vi "Begin.vi"(8 "error in":errorcluster) -> (0 "error out":errorcluster)   [LabVIEW 2019]
doc: "Called before other user functions, this VI is expected to open initial I/O refnums, load in file data, and do all program initialization. Notice that the <B>error out</B> terminal is simply used for data flow. Wiring it to other structures or subVIs ensures that this VI runs first."
uses:
  <vilib>/Rock Robotics/WPI/DriverStation/WPI_DriverStationRobotMode2.ctl
  <vilib>/Rock Robotics/WPI/Joystick/WPI_JoystickDeviceEnum.ctl
  <vilib>/Rock Robotics/SystemInterfaces/DIO/FPGA_DIOPWMChannel.ctl
  <vilib>/Rock Robotics/SystemInterfaces/DIO/FPGA_DIORelayChannel.ctl
  <vilib>/Rock Robotics/WPI/Solenoid/WPI_SolenoidChannel.ctl
  <vilib>/Rock Robotics/SystemInterfaces/DIO/FPGA_DIOChannel.ctl
  <vilib>/Rock Robotics/SystemInterfaces/i2clib/i2c_bus.ctl
  <vilib>/Rock Robotics/SystemInterfaces/AI/FPGA_AIChannel.ctl
  <vilib>/Rock Robotics/SystemInterfaces/spilib/spi_bus.ctl
  Robot Global Data.vi
  <vilib>/Rock Robotics/WPI/MotorControl/WPI_MotorControlOpen SPARK.vi
  <vilib>/Rock Robotics/WPI/MotorControl/WPI_MotorControlOpen Talon.vi
  <vilib>/Rock Robotics/WPI/Solenoid/WPI_SolenoidOpenSingle.vi
  <vilib>/Rock Robotics/WPI/Counter/WPI_CounterDigitalInputToDigitalSource.vi
  Program Files/navX.Library.v2/navX Library v2/IO/Open/Z900_navX_Open_SPI.vi
  Program Files/navX.Library.v2/navX Library v2/navX Library v2.lvlib
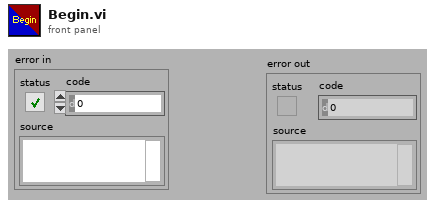
[diagram p1: front panel]
types:
  T1 = typedef "WPI_DriverStationRobotMode2.ctl" = enum16{"Autonomous Disabled", "Autonomous Enabled", "Teleop Disabled", "Teleop Enabled", "Disconnected", "Finish", "Test Disabled", "Test Enabled", "Emergency Stopped"}
  T2 = typedef "WPI_JoystickDeviceEnum.ctl" = enum16{"USB 0", "USB 1", "USB 2", "USB 3", "USB 4", "USB 5"}
  T3 = typedef "WPI_SolenoidChannel.ctl" = enum8{"Solenoid 0", "Solenoid 1", "Solenoid 2", "Solenoid 3", "Solenoid 4", "Solenoid 5", "Solenoid 6", "Solenoid 7", "Invalid"}
  T4 = typedef "FPGA_DIORelayChannel.ctl" = enum8{"Relay 0", "Relay 1", "Relay 2", "Relay 3", "Invalid"}
  T5 = typedef "FPGA_DIOPWMChannel.ctl" = enum8{"PWM 0", "PWM 1", "PWM 2", "PWM 3", "PWM 4", "PWM 5", "PWM 6", "PWM 7", "PWM 8", "PWM 9", "PWM MXP 0", "PWM MXP 1", "PWM MXP 2", "PWM MXP 3", "PWM MXP 4", "PWM MXP 5", "PWM MXP 6", "PWM MXP 7", "PWM MXP 8", "PWM MXP 9", "Invalid"}
  T6 = typedef "FPGA_AIChannel.ctl" = enum8{"AI 0", "AI 1", "AI 2", "AI 3", "AI MXP 0", "AI MXP 1", "AI MXP 2", "AI MXP 3", "Invalid"}
  T7 = typedef "spi_bus.ctl" = enum16{"SPI On-Board, CS0", "SPI On-Board, CS1", "SPI On-Board, CS2", "SPI On-Board, CS3", "SPI MXP", "Invalid"}
  T8 = typedef "i2c_bus.ctl" = enum16{"I2C On-Board", "I2C MXP", "Invalid"}
  T9 = typedef "WPI_CompressorDevRef.ctl" = cluster{"DevStatus":errorcluster, "Pneumatics Control Module":u8}
  T10 = typedef "WPI_JoystickDevRef.ctl" = cluster{"Device":T2}
  T11 = typedef "WPI_MotorControlDeviceRef.ctl" = cluster{"DeviceStatus":errorcluster, "Type":T12, "PWM":cluster{"PWM Channel":T5, "DeadBand":T13}, "CAN":cluster{"Device Number":u8, "SetOutput VI Ref":variant, "GetOutput VI Ref":variant, "Enable VI Ref":variant, "Disable VI Ref":variant, "Data":variant}, "Invert":bool, "DIO PWM":cluster{"PWM \"Enable\" Channel":T5, "DIOChannel":T14, "PWM Rate":dbl}}
  T12 = typedef "WPI_MotorControlType.ctl" = enum16{"PWM", "CAN", "DIO PWM"}
  T13 = typedef "WPI_PWMDeadband.ctl" = cluster{"Name":string, "maxPositivePwm":i32, "minPositivePwm":i32, "centerPwm":i32, "maxNegativePwm":i32, "minNegativePwm":i32, "angularRange":u16}
  T14 = typedef "FPGA_DIOChannel.ctl" = enum8{"DIO 0", "DIO 1", "DIO 2", "DIO 3", "DIO 4", "DIO 5", "DIO 6", "DIO 7", "DIO 8", "DIO 9", "DIO MXP 0", "DIO MXP 1", "DIO MXP 2", "DIO MXP 3", "DIO MXP 4", "DIO MXP 5", "DIO MXP 6", "DIO MXP 7", "DIO MXP 8", "DIO MXP 9", "DIO MXP 10", "DIO MXP 11", "DIO MXP 12", "DIO MXP 13", "DIO MXP 14", "DIO MXP 15", "SPI Port CS1", "SPI Port CS2", "SPI Port CS3", "SPI Port MISO", "SPI Port MOSI", "Invalid"}
  T15 = typedef "WPI_RelayDevRef.ctl" = cluster{"DevStatus":errorcluster, "Relay Channel":T4, "Relay Direction":T16}
  T16 = typedef "WPI_RelayDirection.ctl" = enum16{"Both directions", "Forward only", "Reverse only"}
  T17 = typedef "WPI_SolenoidDevRef.ctl" = cluster{"DevStatus":errorcluster, "Pneumatics Control Module":u8, "Forward Solenoid Channel":T3, "Reverse Solenoid Channel":T3}
  T18 = typedef "WPI_DigitalInputDevRef.ctl" = cluster{"DevStatus":errorcluster, "DIO Channel":T14}
  T19 = typedef "WPI_AnalogChannelDevRef.ctl" = cluster{"DevStatus":errorcluster, "Analog Channel":T6}
  T20 = typedef "navX Library v2.lvlib/Z900_navX_DeviceTypeDef.ctl" = cluster{"Interface":cluster{"Protocol":T21, "Update Rate (4Hz-100Hz)":u8, "navX Open TypeDef":variant}, "Notify Packet":refnum<notifier>, "Loop VI Refnum":refnum<vi>, "Ready to Close Occurrence Refnum":refnum<k4>}
  T21 = typedef "navX Library v2.lvlib/Z900_navX_ProtocolTypeDef.ctl" = enum16{"SERIAL", "I2C", "SPI"}
  T22 = typedef "FPGA_CounterEncoderSourceConvertionLVSourceType.ctl" = cluster{"DevStatus":errorcluster, "AnalogTriggerMode?":bool, "DigitalMode":cluster{"DIO Channel":T23}, "AnalogTriggerMode":cluster{"AnalogTriggerIndex":T24, "OutputType":T25}}
  T23 = typedef "FPGA_DIODigitalSourceChannel.ctl" = enum8{"DIO 0", "DIO 1", "DIO 2", "DIO 3", "DIO 4", "DIO 5", "DIO 6", "DIO 7", "DIO 8", "DIO 9", "DIO MXP 0", "DIO MXP 1", "DIO MXP 2", "DIO MXP 3", "DIO MXP 4", "DIO MXP 5", "DIO MXP 6", "DIO MXP 7", "DIO MXP 8", "DIO MXP 9", "DIO MXP 10", "DIO MXP 11", "DIO MXP 12", "DIO MXP 13", "DIO MXP 14", "DIO MXP 15", "SPI Port CS1", "SPI Port CS2", "SPI Port CS3", "SPI Port MISO", "SPI Port MOSI", "Disabled"}
  T24 = typedef "FPGA_AnalogTriggerIndex.ctl" = enum8{"Trig 0", "Trig 1", "Trig 2", "Trig 3", "Trig 4", "Trig 5", "Trig 6", "Trig 7", "Invalid"}
  T25 = typedef "FPGA_AnalogTriggerOutType.ctl" = enum16{"InWindow", "TriggerState", "Rising", "Falling"}
  T26 = typedef "Color Sensor V3 DevRef.ctl" = cluster{"I2CDevRef":T27}
  T27 = typedef "WPI_I2CDevRef.ctl" = cluster{"DevStatus":errorcluster, "Device Address":u8, "Handle":i32, "I2C Bus":T8}
  T28 = typedef "WPI_EncoderDevRef.ctl" = cluster{"DevStatus":errorcluster, "EncoderIndex":T29, "CounterIndex":T30, "DistancePerCount":dbl, "Decoding Type":T31}
  T29 = typedef "FPGA_EncoderIdx.ctl" = enum8{"Enc 0", "Enc 1", "Enc 2", "Enc 3", "Enc 4", "Enc 5", "Enc 6", "Enc 7", "Invalid"}
  T30 = typedef "FPGA_CounterCtrSystemIndex.ctl" = enum8{"Ctr 0", "Ctr 1", "Ctr 2", "Ctr 3", "Ctr 4", "Ctr 5", "Ctr 6", "Ctr 7", "Invalid"}
  T31 = typedef "WPI_EncoderType.ctl" = enum16{"1x", "2x", "4x"}
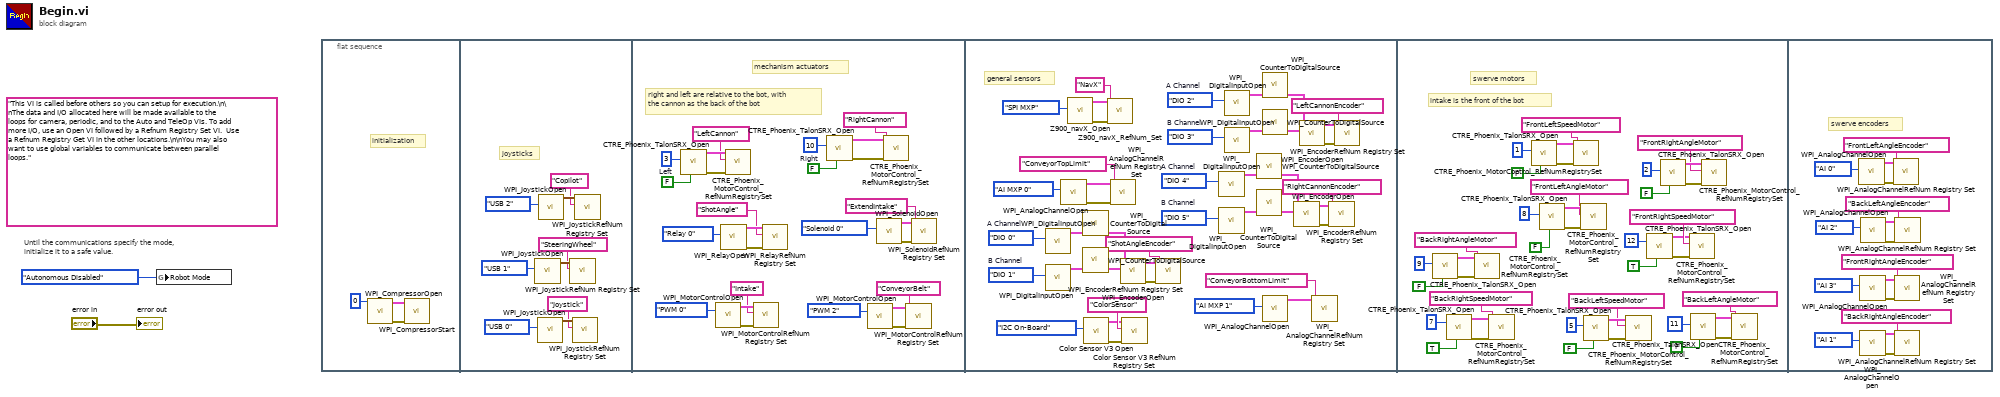
[diagram p0: block diagram]
diagram:
  (unwired) "This VI is called before others so you can setup for execution.\n\nThe data and I/O allocated here will be made available to the loops for camera, periodic, and to the Auto and TeleOp VIs. To add more I/O, use an Open VI followed by a Refnum Registry Set VI.  Use a Refnum Registry Get VI in the other locations.\n\nYou may also want to use global variables to communicate between parallel loops."
  # "Until the communications specify the mode,\ninitialize it to a safe value."
  n1 = global write "Robot Global Data.vi" "Robot Mode"(WPI_DriverStationRobotMode2."Autonomous Disabled" ("Robot Mode")) -> ()
  n2 = flat-sequence {
    frame #0 {
      # "initialization"
      n3 = call <vilib>:"WPI_CompressorOpen.vi"("Pneumatics Control Module (0)"=u8 0) -> ("CompressorDevRef"=w3:T9, "error out"=w5:errorcluster)  [unwired: 13 in]
      n4 = call <vilib>:"WPI_CompressorStart.vi"("error in (no error)"=w5, "CompressorDevRef"=w3) -> ()  [unwired: 8 in, 2 out]
    }
    frame #1 {
      # "joysticks"
      n5 = call <vilib>:"WPI_JoystickOpen.vi"("JoystickDevice"=WPI_JoystickDeviceEnum."USB 1") -> ("JoystickDevRef"=w10:T10)  [unwired: 10 in]
      n6 = call <vilib>:"WPI_JoystickOpen.vi"("JoystickDevice"=WPI_JoystickDeviceEnum."USB 0") -> ("JoystickDevRef"=w11:T10)  [unwired: 10 in]
      n7 = call <vilib>:"WPI_JoystickOpen.vi"("JoystickDevice"=WPI_JoystickDeviceEnum."USB 2") -> ("JoystickDevRef"=w14:T10)  [unwired: 10 in]
      n8 = call <vilib>:"WPI_JoystickRefNum Registry Set.vi"("refnum name"="SteeringWheel", "JoystickDevRef"=w10) -> ()  [unwired: 8 in, 2 out]
      n9 = call <vilib>:"WPI_JoystickRefNum Registry Set.vi"("refnum name"="Joystick", "JoystickDevRef"=w11) -> ()  [unwired: 8 in, 2 out]
      n10 = call <vilib>:"WPI_JoystickRefNum Registry Set.vi"("refnum name"="Copilot", "JoystickDevRef"=w14) -> ()  [unwired: 8 in, 2 out]
    }
    frame #2 {
      w31 = u8 3  # Left
      w32 = u8 10  # Right
      # "right and left are relative to the bot, with\nthe cannon as the back of the bot"
      # "mechanism actuators"
      n11 = call <vilib>:"CTRE_Phoenix_TalonSRX_Open.vi"("Invert"=FALSE, "Device Number"=w31) -> ("error out"=w19:errorcluster, "CAN Talon SRX Ref"=w20:T11)  [unwired: 8 in]
      n12 = call-poly <vilib>:"WPI_MotorControlOpen.vi"("PWM Channel"=FPGA_DIOPWMChannel."PWM 0") -> ("error out"=w40:errorcluster, "MotorControlDeviceRef"=w39:T11)  [unwired: 9 in]
      n13 = call <vilib>:"WPI_RelayOpen.vi"("Relay Channel"=FPGA_DIORelayChannel."Relay 0") -> ("error out"=w30:errorcluster, "RelayDevRef"=w29:T15)  [unwired: 9 in]
      n14 = call <vilib>:"CTRE_Phoenix_MotorControl_RefNumRegistrySet.vi"("error in (no error)"=w19, "refnum name"="LeftCannon", "PhoenixMotorControlDevRef"=w20) -> ()  [unwired: 7 in, 2 out]
      n15 = call <vilib>:"WPI_MotorControlRefNum Registry Set.vi"("error in (no error)"=w40, "refnum name"="Intake", "MotorControlDevRef"=w39) -> ()  [unwired: 7 in, 2 out]
      n16 = call <vilib>:"WPI_RelayRefNum Registry Set.vi"("error in (no error)"=w30, "refnum name"="ShotAngle", "RelayDevRef"=w29) -> ()  [unwired: 7 in, 2 out]
      n17 = call <vilib>:"CTRE_Phoenix_TalonSRX_Open.vi"("Invert"=FALSE, "Device Number"=w32) -> ("error out"=w16:errorcluster, "CAN Talon SRX Ref"=w17:T11)  [unwired: 8 in]
      n18 = call-poly <vilib>:"WPI_MotorControlOpen.vi"("PWM Channel"=FPGA_DIOPWMChannel."PWM 2") -> ("error out"=w36:errorcluster, "MotorControlDeviceRef"=w35:T11)  [unwired: 9 in]
      n19 = call-poly <vilib>:"WPI_SolenoidOpen.vi"("Solenoid Channel"=WPI_SolenoidChannel."Solenoid 0") -> ("error out"=w25:errorcluster, "SolenoidDevRef"=w26:T17)  [unwired: 9 in]
      n20 = call <vilib>:"CTRE_Phoenix_MotorControl_RefNumRegistrySet.vi"("error in (no error)"=w16, "refnum name"="RightCannon", "PhoenixMotorControlDevRef"=w17) -> ()  [unwired: 7 in, 2 out]
      n21 = call <vilib>:"WPI_MotorControlRefNum Registry Set.vi"("error in (no error)"=w36, "refnum name"="ConveyorBelt", "MotorControlDevRef"=w35) -> ()  [unwired: 7 in, 2 out]
      n22 = call <vilib>:"WPI_SolenoidRefNum Registry Set.vi"("error in (no error)"=w25, "refnum name"="ExtendIntake", "SolenoidDevRef"=w26) -> ()  [unwired: 7 in, 2 out]
    }
    frame #3 {
      w52 = FPGA_DIOChannel."DIO 5"  # B Channel
      w51 = FPGA_DIOChannel."DIO 4"  # A Channel
      w61 = FPGA_DIOChannel."DIO 3"  # B Channel
      w60 = FPGA_DIOChannel."DIO 2"  # A Channel
      w82 = FPGA_DIOChannel."DIO 1"  # B Channel
      w81 = FPGA_DIOChannel."DIO 0"  # A Channel
      # "general sensors"
      n23 = call <vilib>:"WPI_DigitalInputOpen.vi"("DIO Channel"=w81) -> ("DigitalInputDevRef"=w78:T18)  [unwired: 1 in, 9 out]
      n24 = call <vilib>:"WPI_DigitalInputOpen.vi"("DIO Channel"=w82) -> ("DigitalInputDevRef"=w79:T18)  [unwired: 1 in, 9 out]
      n25 = call <vilib>:"WPI_AnalogChannelOpen.vi"("Analog Channel"=FPGA_AIChannel."AI MXP 0") -> ("error out"=w68:errorcluster, "AIDeviceRef"=w67:T19)  [unwired: 9 in]
      n26 = call-poly "Z900_navX_Open.vi"("SPI Bus"=spi_bus."SPI MXP") -> ("error out"=w62:errorcluster, "navX Device"=w65:T20)  [unwired: 9 in]
      n27 = call-poly <vilib>:"WPI_CounterToDigitalSource.vi"("DigitalInputDevRef"=w78) -> ("Digital Source"=w77:T22)  [unwired: 6 out]
      n28 = call-poly <vilib>:"WPI_CounterToDigitalSource.vi"("DigitalInputDevRef"=w79) -> ("Digital Source"=w80:T22)  [unwired: 6 out]
      n29 = call <vilib>:"Color Sensor V3 Open.vi"("I2C Bus"=i2c_bus."I2C On-Board") -> ("error out"=w72:errorcluster, "ColorSensorDevRef"=w71:T26)  [unwired: 9 in]
      n30 = call "Z900_navX_RefNum_Set.vi"("error in (no error)"=w62, "refnum name"="NavX", "navX Device"=w65) -> ()  [unwired: 7 in, 2 out]
      n31 = call <vilib>:"WPI_AnalogChannelRefNum Registry Set.vi"("error in (no error)"=w68, "refnum name"="ConveyorTopLimit", "AIDeviceRef"=w67) -> ()  [unwired: 7 in, 2 out]
      n32 = call <vilib>:"WPI_EncoderOpen.vi"("BSource"=w80, "ASource"=w77) -> ("error out"=w76:errorcluster, "EncoderDevRef"=w75:T28)  [unwired: 6 in, 2 out]
      n33 = call <vilib>:"Color Sensor V3 RefNum Registry Set.vi"("error in (no error)"=w72, "refnum name"="ColorSensor", "ColorSensorDevRef"=w71) -> ()  [unwired: 7 in, 2 out]
      n34 = call <vilib>:"WPI_EncoderRefNum Registry Set.vi"("error in (no error)"=w76, "refnum name"="ShotAngleEncoder", "EncoderDevRef"=w75) -> ()  [unwired: 7 in, 2 out]
      n35 = call <vilib>:"WPI_DigitalInputOpen.vi"("DIO Channel"=w51) -> ("DigitalInputDevRef"=w48:T18)  [unwired: 1 in, 9 out]
      n36 = call <vilib>:"WPI_DigitalInputOpen.vi"("DIO Channel"=w52) -> ("DigitalInputDevRef"=w49:T18)  [unwired: 1 in, 9 out]
      n37 = call <vilib>:"WPI_DigitalInputOpen.vi"("DIO Channel"=w60) -> ("DigitalInputDevRef"=w57:T18)  [unwired: 1 in, 9 out]
      n38 = call <vilib>:"WPI_DigitalInputOpen.vi"("DIO Channel"=w61) -> ("DigitalInputDevRef"=w58:T18)  [unwired: 1 in, 9 out]
      n39 = call-poly <vilib>:"WPI_CounterToDigitalSource.vi"("DigitalInputDevRef"=w48) -> ("Digital Source"=w47:T22)  [unwired: 6 out]
      n40 = call-poly <vilib>:"WPI_CounterToDigitalSource.vi"("DigitalInputDevRef"=w49) -> ("Digital Source"=w50:T22)  [unwired: 6 out]
      n41 = call-poly <vilib>:"WPI_CounterToDigitalSource.vi"("DigitalInputDevRef"=w57) -> ("Digital Source"=w56:T22)  [unwired: 6 out]
      n42 = call-poly <vilib>:"WPI_CounterToDigitalSource.vi"("DigitalInputDevRef"=w58) -> ("Digital Source"=w59:T22)  [unwired: 6 out]
      n43 = call <vilib>:"WPI_AnalogChannelOpen.vi"("Analog Channel"=FPGA_AIChannel."AI MXP 1") -> ("AIDeviceRef"=w42:T19)  [unwired: 9 in, 1 out]
      n44 = call <vilib>:"WPI_EncoderOpen.vi"("BSource"=w50, "ASource"=w47) -> ("error out"=w46:errorcluster, "EncoderDevRef"=w45:T28)  [unwired: 6 in, 2 out]
      n45 = call <vilib>:"WPI_EncoderOpen.vi"("BSource"=w59, "ASource"=w56) -> ("error out"=w55:errorcluster, "EncoderDevRef"=w54:T28)  [unwired: 6 in, 2 out]
      n46 = call <vilib>:"WPI_AnalogChannelRefNum Registry Set.vi"("refnum name"="ConveyorBottomLimit", "AIDeviceRef"=w42) -> ()  [unwired: 8 in, 2 out]
      n47 = call <vilib>:"WPI_EncoderRefNum Registry Set.vi"("error in (no error)"=w46, "refnum name"="RightCannonEncoder", "EncoderDevRef"=w45) -> ()  [unwired: 7 in, 2 out]
      n48 = call <vilib>:"WPI_EncoderRefNum Registry Set.vi"("error in (no error)"=w55, "refnum name"="LeftCannonEncoder", "EncoderDevRef"=w54) -> ()  [unwired: 7 in, 2 out]
    }
    frame #4 {
      # "intake is the front of the bot"
      # "swerve motors"
      n49 = call <vilib>:"CTRE_Phoenix_TalonSRX_Open.vi"("Invert"=FALSE, "Device Number"=u8 9) -> ("error out"=w102:errorcluster, "CAN Talon SRX Ref"=w101:T11)  [unwired: 8 in]
      n50 = call <vilib>:"CTRE_Phoenix_TalonSRX_Open.vi"("Invert"=TRUE, "Device Number"=u8 7) -> ("error out"=w117:errorcluster, "CAN Talon SRX Ref"=w118:T11)  [unwired: 8 in]
      n51 = call <vilib>:"CTRE_Phoenix_MotorControl_RefNumRegistrySet.vi"("error in (no error)"=w102, "refnum name"="BackRightAngleMotor", "PhoenixMotorControlDevRef"=w101) -> ()  [unwired: 7 in, 2 out]
      n52 = call <vilib>:"CTRE_Phoenix_MotorControl_RefNumRegistrySet.vi"("error in (no error)"=w117, "refnum name"="BackRightSpeedMotor", "PhoenixMotorControlDevRef"=w118) -> ()  [unwired: 7 in, 2 out]
      n53 = call <vilib>:"CTRE_Phoenix_TalonSRX_Open.vi"("Invert"=FALSE, "Device Number"=u8 1) -> ("error out"=w106:errorcluster, "CAN Talon SRX Ref"=w107:T11)  [unwired: 8 in]
      n54 = call <vilib>:"CTRE_Phoenix_TalonSRX_Open.vi"("Invert"=FALSE, "Device Number"=u8 8) -> ("error out"=w90:errorcluster, "CAN Talon SRX Ref"=w89:T11)  [unwired: 8 in]
      n55 = call <vilib>:"CTRE_Phoenix_MotorControl_RefNumRegistrySet.vi"("error in (no error)"=w106, "refnum name"="FrontLeftSpeedMotor", "PhoenixMotorControlDevRef"=w107) -> ()  [unwired: 7 in, 2 out]
      n56 = call <vilib>:"CTRE_Phoenix_MotorControl_RefNumRegistrySet.vi"("error in (no error)"=w90, "refnum name"="FrontLeftAngleMotor", "PhoenixMotorControlDevRef"=w89) -> ()  [unwired: 7 in, 2 out]
      n57 = call <vilib>:"CTRE_Phoenix_TalonSRX_Open.vi"("Invert"=FALSE, "Device Number"=u8 5) -> ("error out"=w108:errorcluster, "CAN Talon SRX Ref"=w109:T11)  [unwired: 8 in]
      n58 = call <vilib>:"CTRE_Phoenix_MotorControl_RefNumRegistrySet.vi"("error in (no error)"=w108, "refnum name"="BackLeftSpeedMotor", "PhoenixMotorControlDevRef"=w109) -> ()  [unwired: 7 in, 2 out]
      n59 = call <vilib>:"CTRE_Phoenix_TalonSRX_Open.vi"("Invert"=TRUE, "Device Number"=u8 12) -> ("error out"=w115:errorcluster, "CAN Talon SRX Ref"=w116:T11)  [unwired: 8 in]
      n60 = call <vilib>:"CTRE_Phoenix_TalonSRX_Open.vi"("Invert"=FALSE, "Device Number"=u8 2) -> ("error out"=w100:errorcluster, "CAN Talon SRX Ref"=w99:T11)  [unwired: 8 in]
      n61 = call <vilib>:"CTRE_Phoenix_MotorControl_RefNumRegistrySet.vi"("error in (no error)"=w115, "refnum name"="FrontRightSpeedMotor", "PhoenixMotorControlDevRef"=w116) -> ()  [unwired: 7 in, 2 out]
      n62 = call <vilib>:"CTRE_Phoenix_TalonSRX_Open.vi"("Invert"=FALSE, "Device Number"=u8 11) -> ("error out"=w92:errorcluster, "CAN Talon SRX Ref"=w91:T11)  [unwired: 8 in]
      n63 = call <vilib>:"CTRE_Phoenix_MotorControl_RefNumRegistrySet.vi"("error in (no error)"=w100, "refnum name"="FrontRightAngleMotor", "PhoenixMotorControlDevRef"=w99) -> ()  [unwired: 7 in, 2 out]
      n64 = call <vilib>:"CTRE_Phoenix_MotorControl_RefNumRegistrySet.vi"("error in (no error)"=w92, "refnum name"="BackLeftAngleMotor", "PhoenixMotorControlDevRef"=w91) -> ()  [unwired: 7 in, 2 out]
    }
    frame #5 {
      # "swerve encoders"
      n65 = call <vilib>:"WPI_AnalogChannelOpen.vi"("Analog Channel"=FPGA_AIChannel."AI 0") -> ("error out"=w137:errorcluster, "AIDeviceRef"=w138:T19)  [unwired: 9 in]
      n66 = call <vilib>:"WPI_AnalogChannelOpen.vi"("Analog Channel"=FPGA_AIChannel."AI 3") -> ("error out"=w129:errorcluster, "AIDeviceRef"=w130:T19)  [unwired: 9 in]
      n67 = call <vilib>:"WPI_AnalogChannelOpen.vi"("Analog Channel"=FPGA_AIChannel."AI 1") -> ("error out"=w125:errorcluster, "AIDeviceRef"=w126:T19)  [unwired: 9 in]
      n68 = call <vilib>:"WPI_AnalogChannelOpen.vi"("Analog Channel"=FPGA_AIChannel."AI 2") -> ("error out"=w133:errorcluster, "AIDeviceRef"=w134:T19)  [unwired: 9 in]
      n69 = call <vilib>:"WPI_AnalogChannelRefNum Registry Set.vi"("error in (no error)"=w137, "refnum name"="FrontLeftAngleEncoder", "AIDeviceRef"=w138) -> ()  [unwired: 7 in, 2 out]
      n70 = call <vilib>:"WPI_AnalogChannelRefNum Registry Set.vi"("error in (no error)"=w129, "refnum name"="FrontRightAngleEncoder", "AIDeviceRef"=w130) -> ()  [unwired: 7 in, 2 out]
      n71 = call <vilib>:"WPI_AnalogChannelRefNum Registry Set.vi"("error in (no error)"=w125, "refnum name"="BackRightAngleEncoder", "AIDeviceRef"=w126) -> ()  [unwired: 7 in, 2 out]
      n72 = call <vilib>:"WPI_AnalogChannelRefNum Registry Set.vi"("error in (no error)"=w133, "refnum name"="BackLeftAngleEncoder", "AIDeviceRef"=w134) -> ()  [unwired: 7 in, 2 out]
    }
  }
  "error out" <- "error in"
